vi "Process Status Logger.vi"(7 "Action":T1(ring), 8 "error in":errorcluster, 9 "Buffer(lines)":i32=5000, 10 "Log File":path, 11 "Input String":string) -> (0 "error out":errorcluster, 3 "Log":string)   [LabVIEW 2015]
uses:
  Main Globals.vi
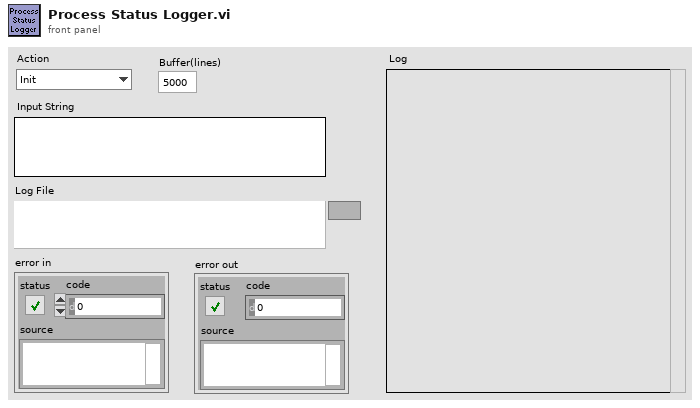
[diagram p1: front panel]
types:
  T1 = enum16{"Init", "Reset", "Read", "Update", "Close"}
  T2 = enum16{"open", "replace", "create", "open or create", "replace or create", "replace or create with confirmation"}
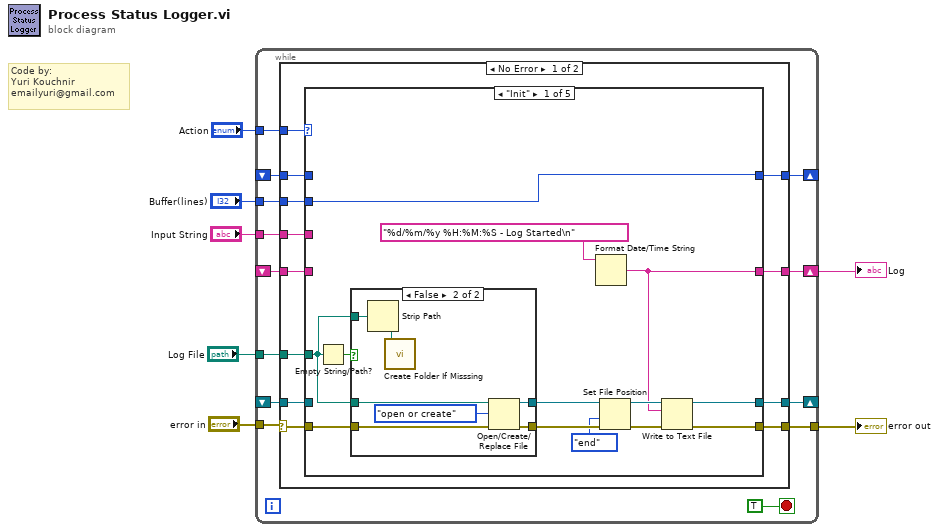
[diagram p0: block diagram]
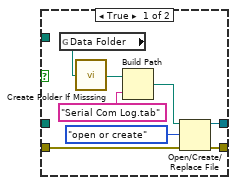
[diagram p2: hidden frame]
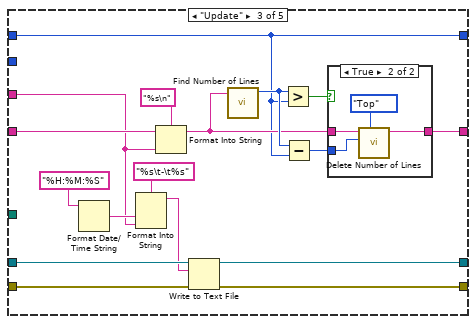
[diagram p4: hidden frame]
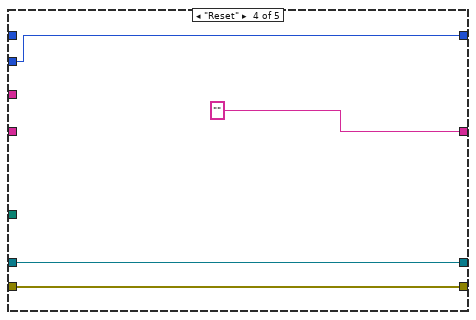
[diagram p6: hidden frame]
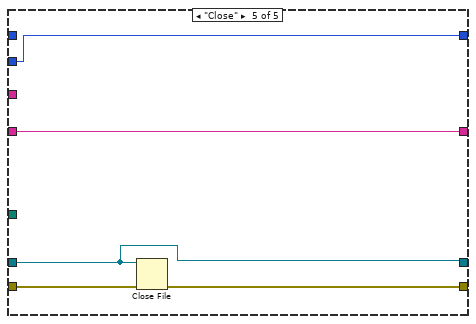
[diagram p7: hidden frame]
diagram:
  # "Code by:\nYuri Kouchnir\nemailyuri@gmail.com"
  n1 = while {
    tunnel: "error in" -> [w19]
    tunnel: [w15] -> w6
    tunnel: "Action" -> [w18]
    tunnel: "Log File" -> [w17]
    tunnel: "Input String" -> [w16]
    shift-right: [w14] -> _
    shift-left: _ -> [w13]
    shift-right: [w12] -> w2
    shift-left: _ -> [w11]
    shift-right: [w10] -> _
    shift-left: _ -> [w9]
    tunnel: "Buffer(lines)" -> [w8]
    stop <- TRUE stop-if-true
    n2 = case shown="No Error" w19 {
      selector: w19 -> [w32 w98]
      tunnel: w18 -> [w31 _]
      tunnel: w17 -> [w30 _]
      tunnel: w16 -> [w29 _]
      tunnel: [w28 w98] -> w15
      tunnel: [w27 w99] -> w14
      tunnel: w13 -> [w26 w99]
      tunnel: [w25 w97] -> w12
      tunnel: w11 -> [w24 w97]
      tunnel: w9 -> [w23 w96]
      tunnel: [w22 w96] -> w10
      tunnel: w8 -> [w21 _]
      frame No Error {
        n3 = case shown="\"Init\"" w31 {
          tunnel: w32 -> [w44 w63 w81 w88 w94]
          tunnel: w30 -> [w43 _ _ _ _]
          tunnel: w29 -> [_ _ w68 _ _]
          tunnel: [w37 w63 w66 w88 w93] -> w28
          tunnel: [w36 w62 w67 w89 w92] -> w27
          tunnel: w26 -> [_ w62 w77 w89 w92]
          tunnel: [w34 w64 w70 "" ("Resulting String") w95] -> w25
          tunnel: w24 -> [_ w64 w75 _ w95]
          tunnel: w23 -> [_ _ w65 _ _]
          tunnel: [w33 w61 w65 w87 w91] -> w22
          tunnel: w21 -> [w33 w61 _ w87 w91]
          frame "Init" {
            n4 = Empty String/Path?(string/path=w43) -> (empty?=w45:bool)
            n5 = case shown="False" w45 {
              tunnel: w44 -> [w48 w59]
              tunnel: [w47 w58] -> w42
              tunnel: w43 -> [_ w56]
              tunnel: w43 -> [_ w55]
              tunnel: [w46 w54] -> w41
              frame True {
                n6 = global read "Main Globals.vi" "Data Folder"() -> (w53:path)
                n7 = call "Create Folder If Misssing.vi"("Path In"=w53) -> ("Path Out"=w52:path)
                n8 = Build Path(base path=w52, name or relative path="Serial Com Log.tab") -> (appended path=w50:path)
                n9 = Open/Create/Replace File(file path (use dialog)=w50, error in=w48, operation (0:open)=T2."open or create") -> (refnum out=w46:refnum<file>, error out=w47:errorcluster)  [unwired: 3 in, 1 out]
              }
              frame False {
                n10 = Strip Path(path=w56) -> (stripped path=w57:path)  [unwired: 1 out]
                n11 = call "Create Folder If Misssing.vi"("Path In"=w57) -> ()  [unwired: 1 out]
                n12 = Open/Create/Replace File(file path (use dialog)=w55, error in=w59, operation (0:open)=T2."open or create") -> (refnum out=w54:refnum<file>, error out=w58:errorcluster)  [unwired: 3 in, 1 out]
              }
            }
            n13 = Format Date/Time String(time format string (%c)="%d/%m/%y %H:%M:%S - Log Started\n") -> (date/time string=w34:string)  [unwired: 2 in]
            n14 = Set File Position(refnum=w41, from (0:start)=enum16{"start", "end", "current"}."end", error in=w42) -> (refnum out=w39:refnum<file>, error out=w35:errorcluster)  [unwired: 1 in]
            n15 = Write to Text File(file (use dialog)=w39, text=w34, error in=w35) -> (refnum out=w36:refnum<file>, error out=w37:errorcluster)  [unwired: 1 in, 1 out]
          }
          frame "Read" {
          }
          frame "Update" {
            n16 = Format Date/Time String(time format string (%c)="%H:%M:%S") -> (date/time string=w78:string)  [unwired: 2 in]
            n17 = Format Into String(format string="%s\t-\t%s", w78, w68) -> (resulting string=w76:string)  [unwired: 2 in, 1 out]
            n18 = Format Into String(format string="%s\n", initial string=w75, w68) -> (resulting string=w71:string)  [unwired: 1 in, 1 out]
            n19 = Write to Text File(file (use dialog)=w77, text=w76, error in=w81) -> (refnum out=w67:refnum<file>, error out=w66:errorcluster)  [unwired: 1 in, 1 out]
            n20 = call "Find Number of Lines.vi"("String"=w71) -> ("Number of Lines"=w73:i32)  [unwired: 10 in]
            n21 = Greater?(x=w73, y=w65) -> (0:w74:bool)
            n22 = Subtract(x=w73, y=w65) -> (x-y=w72:i32)
            n23 = case shown="True" w74 {
              tunnel: w72 -> [_ w85]
              tunnel: w71 -> [w82 w86]
              tunnel: [w82 w84] -> w70
              frame False {
              }
              frame True {
                n24 = call "Delete Number of Lines.vi"("Position"=enum16{"Top", "Bottom", "Line N"}."Top", "Number of Lines"=w85, "String"=w86) -> ("Resulting String"=w84:string)  [unwired: 8 in]
              }
            }
          }
          frame "Reset" {
          }
          frame "Close" {
            n25 = Close File(refnum=w92, error in=w94) -> (error out=w93:errorcluster)  [unwired: 1 out]
          }
        }
      }
      frame Error {
      }
    }
  }
  "error out" <- w6
  "Log" <- w2
